vi "运行状态时间点索引.vi"(10 "索引":i32) -> (2 "数值":dbl)   [LabVIEW 2020]
uses:
  Global.vi
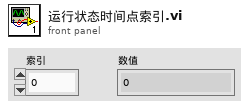
[diagram p1: front panel]
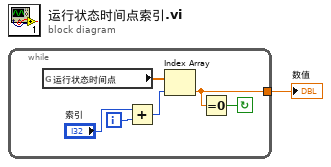
[diagram p0: block diagram]
diagram:
  n1 = while {
    tunnel: [w2] -> w1
    i -> [w5]
    stop <- w3 continue-if-true
    n2 = global read "Global.vi" "运行状态时间点"() -> (w7:dbl[])
    n3 = Add(x="索引", y=w5) -> (x+y=w4:i32)
    n4 = Index Array(array=w7, index=w4) -> (element=w2:dbl)
    n5 = Equal To 0?(x=w2) -> (x = 0?=w3:bool)
  }
  "数值" <- w1
